vi "add-br-.vi"   [LabVIEW 2018]
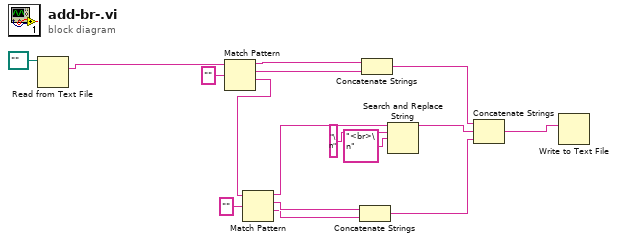
[diagram p0: block diagram]
diagram:
  n1 = Read from Text File(file (use dialog)=path "") -> (text=w15:string)  [unwired: 3 in, 3 out]
  n2 = Match Pattern(string=w15, regular expression="") -> (before substring=w12:string, match substring=w11:string, after substring=w6:string)  [unwired: 1 in, 1 out]
  n3 = Match Pattern(string=w6, regular expression="") -> (before substring=w5:string, match substring=w10:string, after substring=w9:string)  [unwired: 1 in, 1 out]
  n4 = Concatenate Strings(w10, w9) -> (w7:string)
  n5 = Concatenate Strings(w12, w11) -> (w8:string)
  n6 = Search and Replace String(input string=w5, search string="\n", replace string="<br>\n" ("replace string (\"\")")) -> (result string=w2:string)  [unwired: 5 in, 3 out]
  n7 = Concatenate Strings(w8, w2, w7) -> (w1:string)
  n8 = Write to Text File(text=w1) -> ()  [unwired: 3 in, 3 out]
